vi "Create Body.vi"(8 "error in (no error)":errorcluster, 11 "Body Parameters":T1[](array[typedef])) -> (0 "error out":errorcluster, 3 "Body":string)   [LabVIEW 2011, in "i3-oauth.lvlib"]
doc: "Use this template to build a VI to use as a subVI."
uses:
  i3-oauth.lvlib
  Controls/Name-Value Pair.ctl
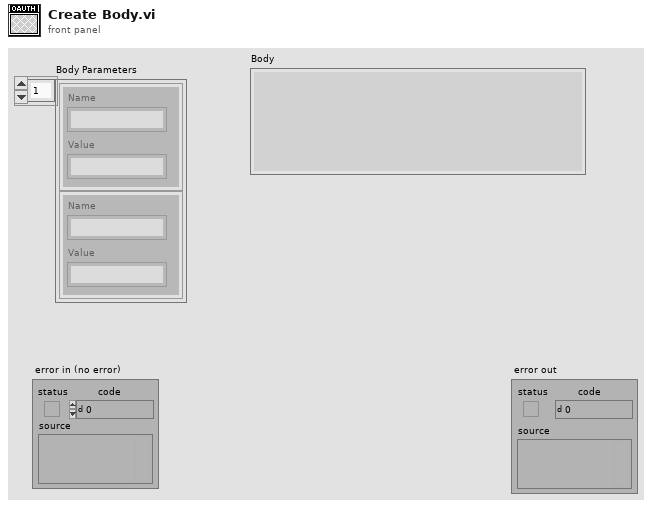
[diagram p1: front panel]
types:
  T1 = typedef "i3-oauth.lvlib/Name-Value Pair.ctl" = cluster{"Name":string, "Value":string}
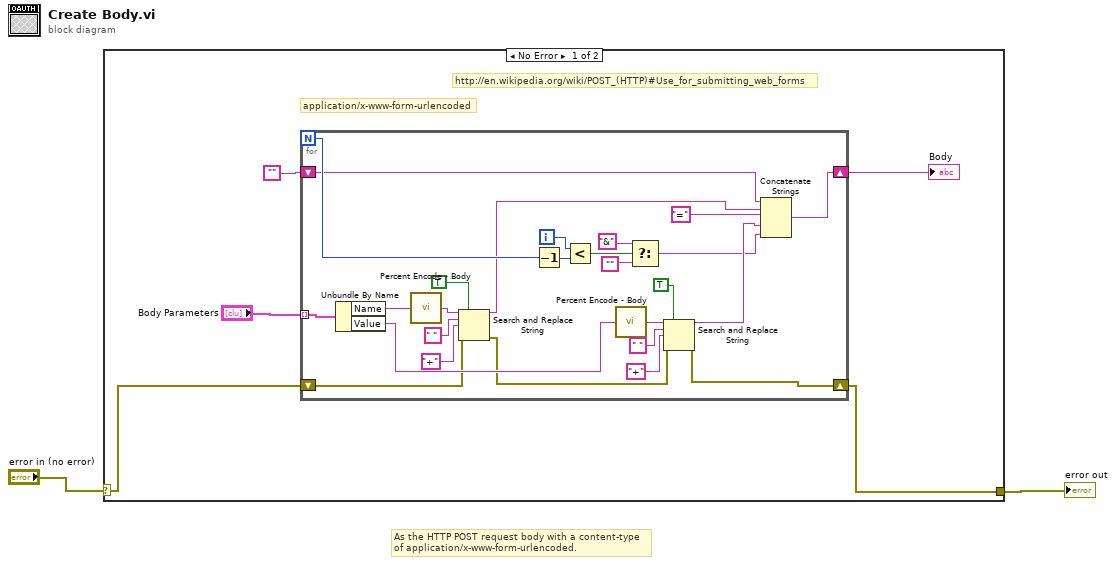
[diagram p0: block diagram]
diagram:
  # "As the HTTP POST request body with a content-type \nof application/x-www-form-urlencoded."
  n1 = case shown="No Error" "error in (no error)" {
    selector: "error in (no error)" -> [w4 w34]
    tunnel: [w3 w34] -> w1
    frame No Error {
      # "application/x-www-form-urlencoded"
      # "http://en.wikipedia.org/wiki/POST_(HTTP)#Use_for_submitting_web_forms"
      n2 = for {
        N -> [w29]
        shift-right: [w31] -> w6
        shift-left: "" -> [w16]
        tunnel: "Body Parameters" -> [w33] mode=indexing
        shift-right: [w9] -> w3
        shift-left: w4 -> [w11]
        i -> [w30]
        n3 = Unbundle By Name(w33) -> ("Name"=w17:string, "Value"=w15:string)
        n4 = call "Percent Encode - Body.vi"("unescaped string in"=w17) -> ("escaped string out"=w18:string)
        n5 = Search and Replace String(replace all?=TRUE ("replace all? (F)"), input string=w18, search string=" ", replace string="+" ("replace string (\"\")"), error in=w11) -> (result string=w8:string, error out=w10:errorcluster)  [unwired: 3 in, 2 out]
        n6 = Decrement(x=w29) -> (x-1=w28:i32)
        n7 = Less?(x=w30, y=w28) -> (x < y?=w27:bool)
        n8 = call "Percent Encode - Body.vi"("unescaped string in"=w15) -> ("escaped string out"=w14:string)
        n9 = Select(t="&", s=w27, f="") -> (s? t:f=w13:string)
        n10 = Search and Replace String(replace all?=TRUE ("replace all? (F)"), input string=w14, search string=" ", replace string="+" ("replace string (\"\")"), error in=w10) -> (result string=w19:string, error out=w9:errorcluster)  [unwired: 3 in, 2 out]
        n11 = Concatenate Strings(w16, w8, "=" ("string"), w19, w13) -> (w31:string)
      }
      "Body" <- w6
    }
    frame Error {
    }
  }
  "error out" <- w1
